vi "XLP80_Globals_Action.vi"() -> ()   [LabVIEW 2021]
uses:
  XLP80_Action/XLP80_Action_TDefCluster_DCDC.ctl
panel:
  in  "Server":T1(tab)
  out "Server HH":bool=TRUE
  out "Server HH OK":bool=TRUE
  out "Server EA OK":bool
  out "Server EA":bool
  out "Server EIP OK":bool
  out "Server EIP":bool
  out "Server State OK":bool=TRUE
  out "Server State":bool=TRUE
  out "Server Datalog OK":bool=TRUE
  out "Server Datalog":bool=TRUE
  in  "CycleCalcSet":u32=100
  out "Server Output OK":bool=TRUE
  out "Server Output":bool=TRUE
  out "Server CAN OK":bool
  out "Server CAN":bool
  in  "CycleTimeCAN":i32
  in  "Debug_DI":bool[](array[boolean])
  in  "Debug_AI":sgl[](array[numeric])
  in  "Debug_CAN ReaD":dbl[](array[numeric])
  in  "Logic DCDC":T2 {"t_71_Iout" format="%.1f s"; "t_71_Uout" format="%.1f s"; "t_71_Uin" format="%.1f s"; "71_Iout_Soll2" format="%.1f A"; "71_Iout_Soll1" format="%.1f A"; "71_Uout_Soll2" format="%.1f V"; "71_Uout_Soll1" format="%.1f V"; "71_Uin_Soll2" format="%.1f V"; "71_Uin_Soll1" format="%.1f V"}
  in  "but_back_NormalOperation":bool
  in  "but_next_NormalOperation":bool
  in  "but_ResetShutdown":bool
  in  "Alarm":bool
  in  "but_ResetAlarm":bool
  in  "but_back_Power Management":bool
  in  "but_next_Power Management":bool
  in  "but_next_Basis Funktion":bool
  in  "but_back_Basis Funktion":bool
  in  "but_next_HV & Software":bool
  in  "Set System Off":bool
  out "Profile_actTime":sgl
  out "Profile_TotalTime":sgl
  in  "Shutdown":bool
  in  "ResetError":bool
  in  "Off":bool
  in  "Interval":i32
  in  "Save":bool caption="Read object configuration"
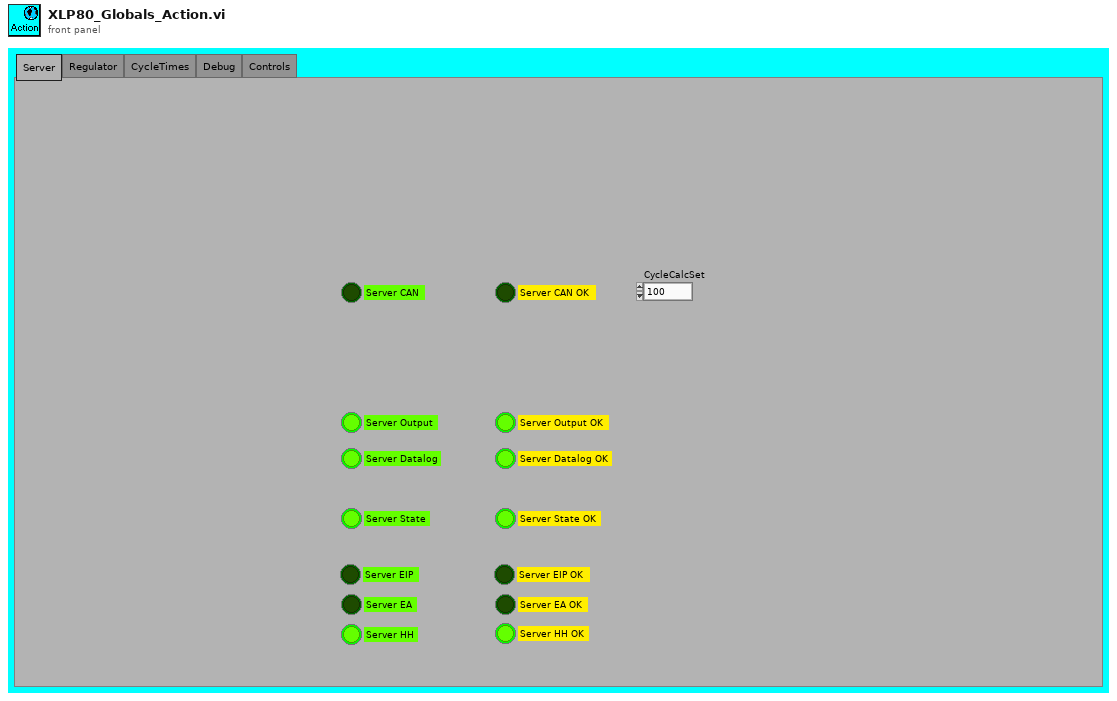
[diagram p1: front panel]
types:
  T1 = enum32{"Server", "Regulator", "CycleTimes", "Debug", "Controls"}
  T2 = typedef "XLP80_Action_TDefCluster_DCDC.ctl" = cluster{"71_Uin_Soll1":dbl, "71_Uin_Soll2":dbl, "t_71_Uin":dbl, "71_Uout_Soll1":dbl, "71_Uout_Soll2":dbl, "t_71_Uout":dbl, "71_Iout_Soll1":dbl, "71_Iout_Soll2":dbl, "t_71_Iout":dbl, "Logic Enable":bool}
diagram:
